vi "ExSimpleAsyncNIDisplayGbl.vi"() -> ()   [LabVIEW 2010]
uses:
  Open-Close Hardware/CamHandle.vi
panel:
  out "Image Display":u16[][](graph)
  in  "Timing Mode":u32(ring)=1 items=["N/A", "Free Run/Timed", "Trigger First (PM only)", "Ext Sync/Strobed ", "Variable Exp (PM only)", "Flash Mode (PM only)"]
  in  "Exposure":dbl min=0.0 step=0.001 format="%.3f"
  in  "stop":bool
  out "error out":errorcluster
  in  "error in (no error)":errorcluster
  # "ExSimipleAsyncNIDisplay:\nThis is a Full Frame Async example, using NI image display. This should work with \nall camera systems. It requires a start for every frame collected. Not all timing modes \nwork for all cameras, also the trigger edge only applies to Princeton Instrument \ncameras. Not all cameras have the ability to set the temperature.\nPressing the stop button stops the example."
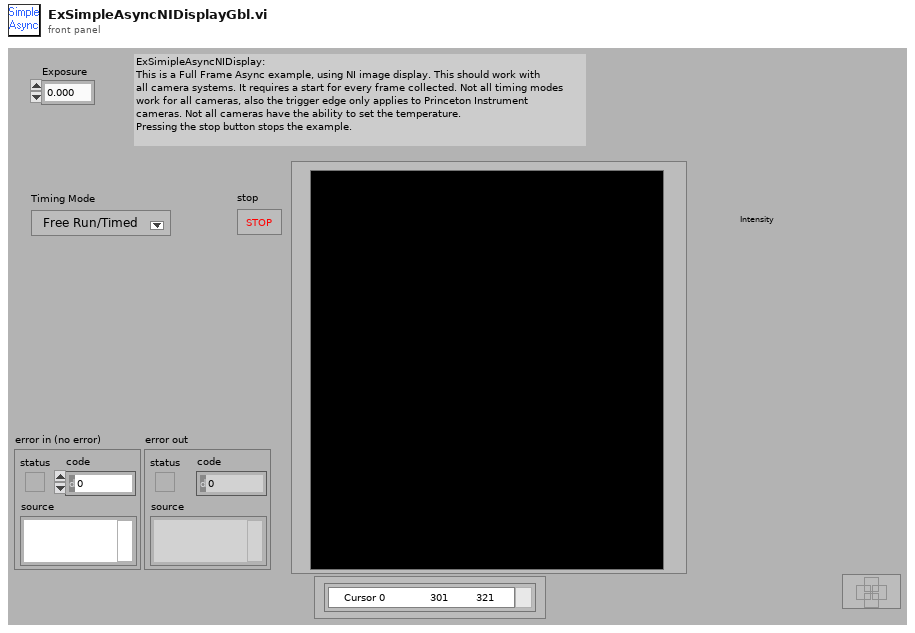
[diagram p1: front panel]
types:
  T1 = cluster{"Acquire mode \n3 is Async":i32, "Exposure":dbl, "Number of Images":i32, "Software Accums":i32}
  T2 = cluster{"Camera Handle":u32, "Pulser Handle":u32, "File Handle":u32, "Display Handle":u32, "Image Handle":u32}
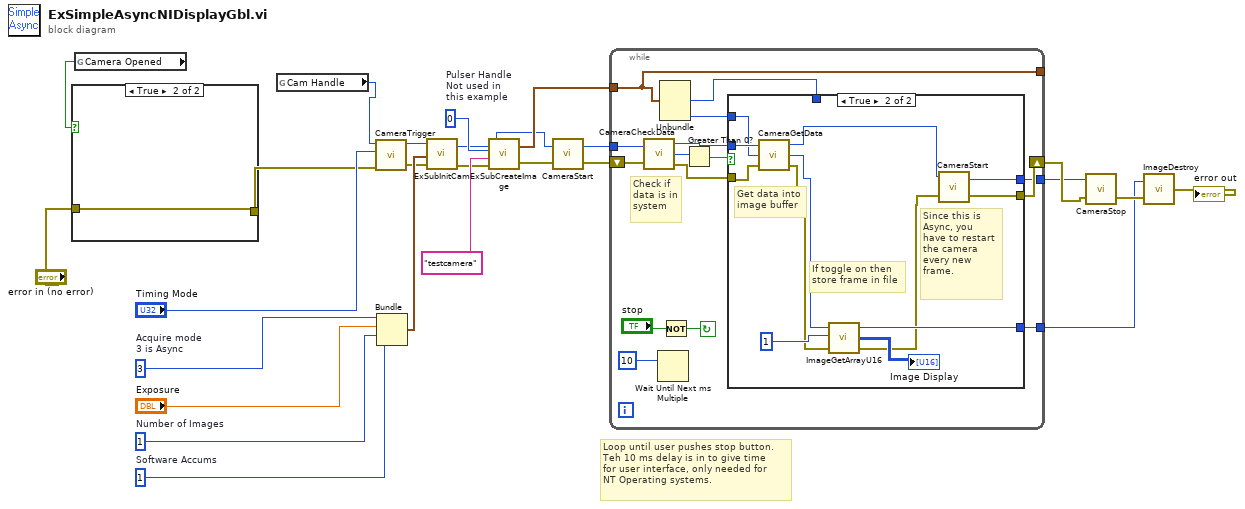
[diagram p0: block diagram]
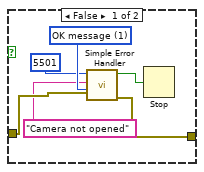
[diagram p2: hidden frame]
diagram:
  w18 = 0  # Pulser Handle Not used in  this example
  w23 = 1  # Number of Images
  w24 = 3  # Acquire mode  3 is Async
  w22 = 1  # Software Accums
  # "Loop until user pushes stop button.\nTeh 10 ms delay is in to give time \nfor user interface, only needed for \nNT Operating systems."
  n1 = global read "CamHandle.vi" "Camera Opened"() -> (w9:bool)
  n2 = case shown="True" w9 {
    tunnel: "error in (no error)" -> [w30 w32]
    tunnel: [w29 w32] -> w7
    frame False {
      w31 = u16 1 items=["no dialog", "OK message", "continue or stop message"] ("type of dialog (OK msg:1)")
      n3 = call <vilib>:"Simple Error Handler.vi"("error code (no error:0)"=5501, "error source (\" \")"="Camera not opened", "type of dialog (OK msg:1)"=w31, "error in (no error)"=w30) -> ("error?"=w27:bool, "error out"=w29:errorcluster)  [unwired: 1 in, 3 out]
      n4 = Stop(stop? (T)=w27) -> ()
    }
    frame True {
    }
  }
  n5 = global read "CamHandle.vi" "Cam Handle"() -> (w8:u32)
  n6 = call <userlib>:"CameraTrigger.vi"("error in"=w7, "Timing Mode"="Timing Mode", "Camera Handle"=w8) -> ("error out"=w13:errorcluster, "Camera Handle"=w12:u32)  [unwired: 1 in]
  n7 = Bundle("Acquire mode \n3 is Async"=w24, "Exposure"="Exposure", "Number of Images"=w23, "Software Accums"=w22) -> (w20:T1)  [unwired: 1 in]
  n8 = call "ExSubInitCam.vi"("error in (no error)"=w13, "Camera Information"=w20, "Camera Handle"=w12) -> ("error out"=w19:errorcluster, "Camera Handle"=w15:u32)
  n9 = call "ExSubCreateImage.vi"("error in (no error)"=w19, "File and Display Name"="testcamera", "Pulser Handle"=w18, "Camera Handle"=w15) -> ("error out"=w17:errorcluster, "Handles Out"=w16:T2)
  n10 = call <userlib>:"CameraStart.vi"("error in"=w17, "Camera Handle"=w15) -> ("error out"=w10:errorcluster, "Camera Handle"=w11:u32)
  n11 = while {
    tunnel: w16 -> [w35]
    tunnel: w11 -> [w44]
    shift-right: [w38] -> w5
    shift-left: w10 -> [w39]
    tunnel: [w35] -> _
    tunnel: [w34] -> w2
    tunnel: [w33] -> w1
    stop <- w46 continue-if-true
    # "Check if \ndata is in\nsystem"
    n12 = call <userlib>:"CameraCheckData.vi"("Camera Handle"=w44, "error in"=w39) -> ("Camera Handle"=w41:u32, "Number Of Frames Available"=w43:i32, "error out"=w40:errorcluster)
    n13 = Wait Until Next ms Multiple(millisecond multiple=10) -> ()  [unwired: 1 out]
    n14 = Unbundle(w35) -> ("File Handle"=w37:u32, "Image Handle"=w36:u32)  [unwired: 3 out]
    n15 = Not(x="stop") -> (.not. x?=w46:bool)
    n16 = Greater Than 0?(x=w43) -> (x > 0?=w42:bool)
    n17 = case shown="True" w42 {
      tunnel: w41 -> [w49 w62]
      tunnel: w40 -> [w50 w61]
      tunnel: w37 -> [_ _]
      tunnel: [w50 w59] -> w38
      tunnel: w36 -> [w48 w54]
      tunnel: [w49 w53] -> w34
      tunnel: [w48 w52] -> w33
      frame False {
      }
      frame True {
        # "If toggle on then\nstore frame in file"
        # "Since this is \nAsync, you\nhave to restart \nthe camera\nevery new \nframe."
        # "Get data into\nimage buffer"
        n18 = call <userlib>:"CameraGetData.vi"("error in"=w61, "Data Handle"=w54, "Camera Handle"=w62) -> ("error out"=w55:errorcluster, "Data Handle"=w57:u32, "Camera Handle"=w60:u32)
        n19 = call <userlib>:"ImageGetArrayU16.vi"("error in"=w55, "Z position"=1, "Image Handle"=w57) -> ("error out"=w51:errorcluster, "Array uint 16"=→"Image Display":u16[][], "Image Handle"=w52:u32)
        n20 = call <userlib>:"CameraStart.vi"("error in"=w51, "Camera Handle"=w60) -> ("error out"=w59:errorcluster, "Camera Handle"=w53:u32)
      }
    }
  }
  n21 = call <userlib>:"CameraStop.vi"("error in"=w5, "Camera Handle"=w2) -> ("error out"=w4:errorcluster)  [unwired: 1 out]
  n22 = call <userlib>:"ImageDestroy.vi"("error in"=w4, "Data handle"=w1) -> ("error out"=→"error out":errorcluster)
